vi "init_delay_generator.vi"(4 "reset TRIG":bool, 8 "VISA resource name":refnum<visa-resource-name>="TRIG") -> (0 "error out":errorcluster, 3 "VISA resource name out":refnum<visa-resource-name>)   [LabVIEW 2011]
doc: "Initializes the delay generator to the defaults settings, leaves the delay data untouched."
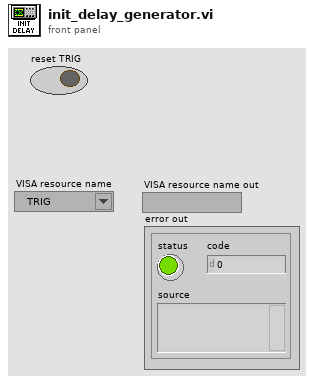
[diagram p1: front panel]
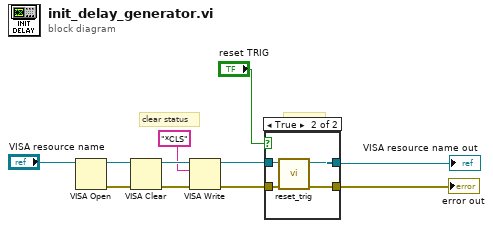
[diagram p0: block diagram]
diagram:
  # "RESET"
  # "clear status"
  n1 = VISA Open(VISA resource name="VISA resource name") -> (VISA resource name=w10:refnum<visa-resource-name>, error out=w11:errorcluster)  [unwired: 4 in]
  n2 = VISA Clear(VISA resource name=w10, error in (no error)=w11) -> (VISA resource name out=w9:refnum<visa-resource-name>, error out=w8:errorcluster)
  n3 = VISA Write(VISA resource name=w9, write buffer="*CLS" ("Query 2"), error in (no error)=w8) -> (VISA resource name out=w5:refnum<visa-resource-name>, error out=w4:errorcluster)  [unwired: 1 out]
  n4 = case shown="True" "reset TRIG" {
    tunnel: w5 -> [w13 w17]
    tunnel: w4 -> [w12 w16]
    tunnel: [w13 w14] -> w3
    tunnel: [w12 w15] -> w2
    frame False {
    }
    frame True {
      n5 = call "reset_trig.vi"("error in (no error)"=w16, "VISA resource name"=w17) -> ("error out"=w15:errorcluster, "VISA resource name out"=w14:refnum<visa-resource-name>)  [unwired: 8 in]
    }
  }
  "VISA resource name out" <- w3
  "error out" <- w2
